vi "Data.vi"(8 "error in (no error)":errorcluster caption="entrée d'erreur (pas d'erreur)", 11 "Load_Boston en entrée":refnum<class "Load_Boston.lvclass">) -> (0 "error out":errorcluster caption="sortie d'erreur", 3 "Load_Boston en sortie":refnum<class "Load_Boston.lvclass">)   [LabVIEW 2020, in "Load_Boston.lvclass"]
uses:
  Load_Boston.lvclass
  Load_Boston.lvclass/Load_Boston.ctl
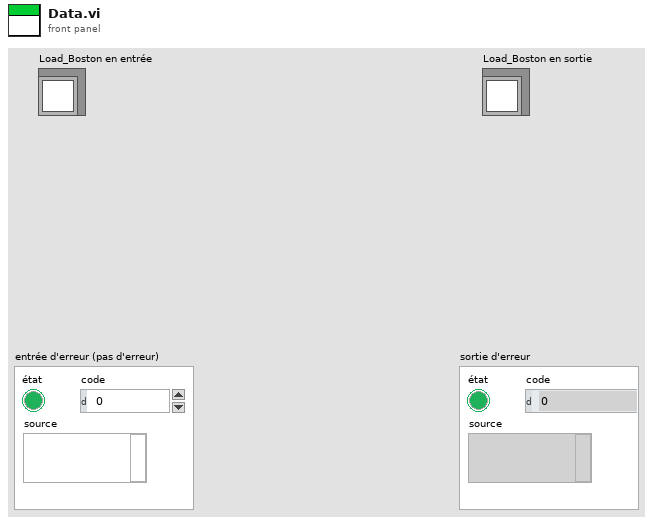
[diagram p1: front panel]
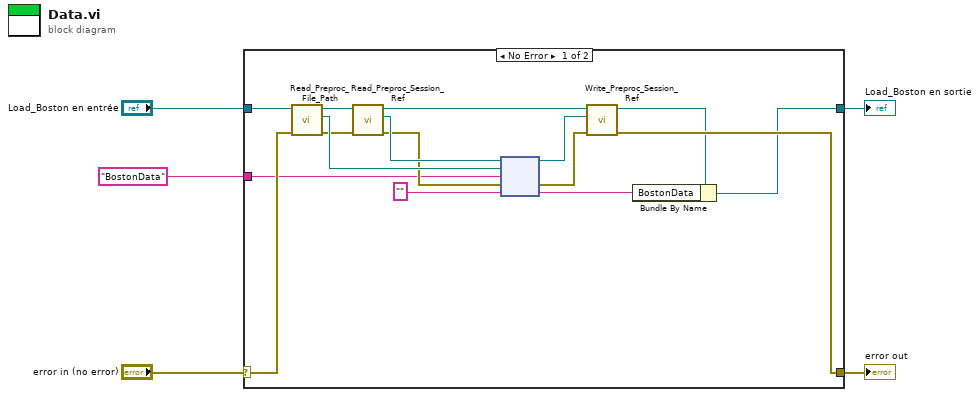
[diagram p0: block diagram]
diagram:
  n1 = case shown="No Error" "error in (no error)" {
    selector: "error in (no error)" -> [w11 w23]
    tunnel: [w10 w23] -> w4
    tunnel: [w7 w22] -> w2
    tunnel: "Load_Boston en entrée" -> [w12 w22]
    tunnel: "BostonData" -> [w9 _]
    frame No Error {
      n2 = call-dynamic "Read_Preproc_File_Path.vi"("error in (no error)"=w11, "Python in"=w12) -> ("error out"=w16:errorcluster, "File_Path"=w19:path, "Python out"=w21:refnum<class "Load_Boston.lvclass">)  [unwired: 7 in]
      n3 = call-dynamic "Read_Preproc_Session_Ref.vi"("error in (no error)"=w16, "Python in"=w21) -> ("error out"=w17:errorcluster, "Session_ref"=w18:refnum<k35>, "Python out"=w20:refnum<class "Load_Boston.lvclass">)  [unwired: 7 in]
      n4 = node(w18, w19, w9, w17, "") -> (w13:refnum<k35>, w15:errorcluster, w6:string)  [unwired: 2 out]
      n5 = call-dynamic "Write_Preproc_Session_Ref.vi"("error in (no error)"=w15, "Session_ref"=w13, "Python in"=w20) -> ("error out"=w10:errorcluster, "Python out"=w8:refnum<class "Load_Boston.lvclass">)  [unwired: 7 in]
      n6 = Bundle By Name(cluster=w8, "BostonData"=w6) -> (w7:refnum<class "Load_Boston.lvclass">)
    }
    frame Error {
    }
  }
  "error out" <- w4
  "Load_Boston en sortie" <- w2
